vi "Dl-to-pos.vi"(2 "DL param":cluster{"min":dbl, "max":dbl, "real pos":dbl}, 3 "DL_pos":dbl) -> (0 "pos, mm":dbl, 1 "DL pos":dbl)   [LabVIEW 2020, in "OWIS_DLs_h.xctl"]
uses:
  OWIS_DLs_h.xctl
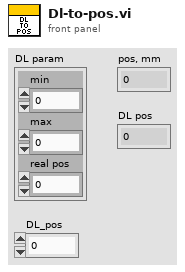
[diagram p1: front panel]
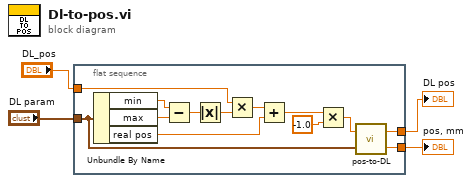
[diagram p0: block diagram]
diagram:
  n1 = flat-sequence {
    tunnel: "DL param" -> [w8]
    tunnel: "DL_pos" -> [w6]
    tunnel: [w7] -> w2
    tunnel: [w5] -> w1
    frame #0 {
      n2 = Unbundle By Name(w8) -> ("min"=w10:dbl, "max"=w11:dbl, "real pos"=w17:dbl)
      n3 = Subtract(x=w10, y=w11) -> (x-y=w15:dbl)
      n4 = Absolute Value(x=w15) -> (abs(x)=w14:dbl)
      n5 = Multiply(x=w6, y=w14) -> (x*y=w16:dbl)
      n6 = Add(x=w16, y=w17) -> (x+y=w13:dbl)
      n7 = Multiply(x=w13, y=-1.0) -> (x*y=w9:dbl)
      n8 = call "pos-to-DL.vi"("DL param"=w8, "pos, mm"=w9) -> ("pos, mm"=w7:dbl, "DL pos"=w5:dbl)
    }
  }
  "DL pos" <- w1
  "pos, mm" <- w2
